vi "CorrectInvalidProfile.vi"(0 "v0x":dbl, 1 "s3x":dbl, 2 "s0x":dbl, 3 "a1":dbl, 4 "index":i32, 5 "v3x":dbl, 7 "Path  Smooth":dbl[][](array[numeric]), 9 "v3y":dbl, 11 "v0y":dbl, 12 "s3y":dbl, 13 "s0y":dbl, 14 "a3":dbl) -> (6 "New v3x":dbl, 10 "New v3y":dbl)   [LabVIEW 2018]
uses:
  <vilib>/Analysis/coordinate.llb/Wrap Angle (scalar).vi
  <vilib>/Analysis/_algsub.llb/Real Vector Norm.vi
  <vilib>/Analysis/NI_AAL_Angle.lvlib
  <vilib>/Analysis/NI_AALPro.lvlib
panel:
  out "v3x 2":dbl
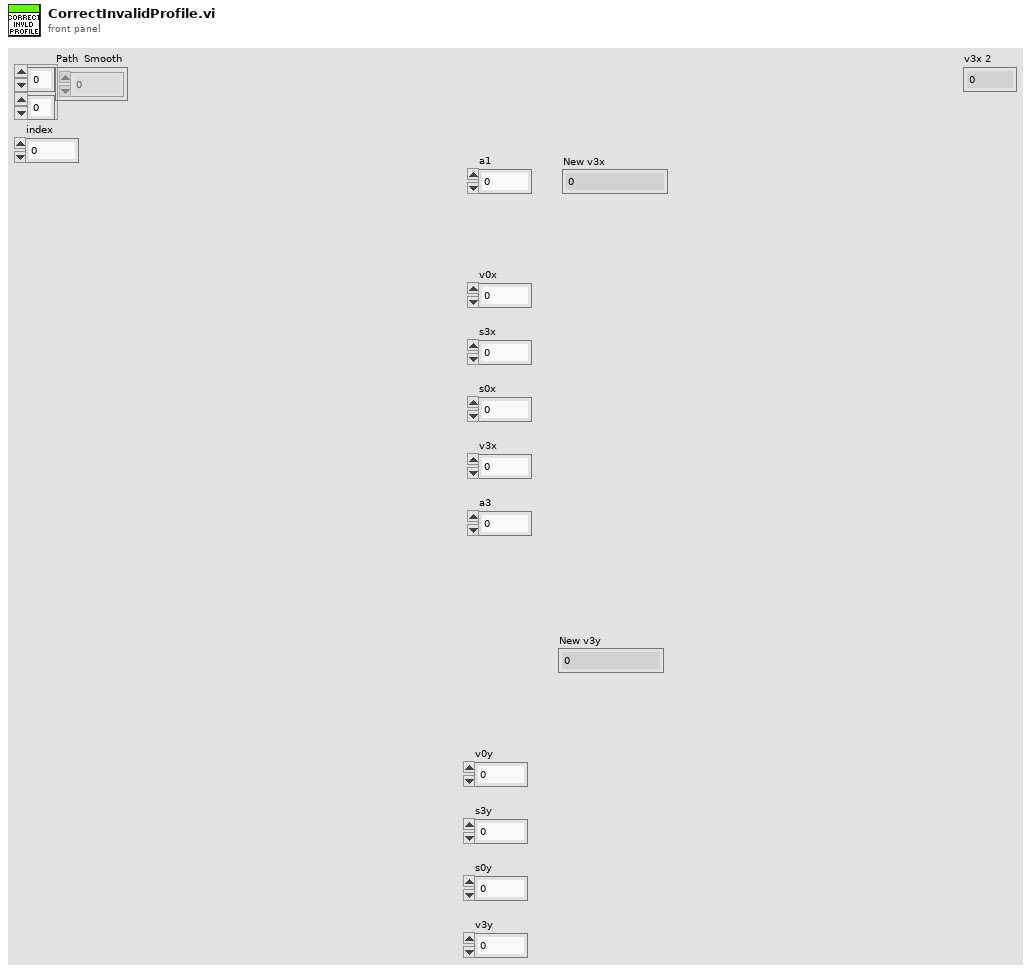
[diagram p1: front panel]
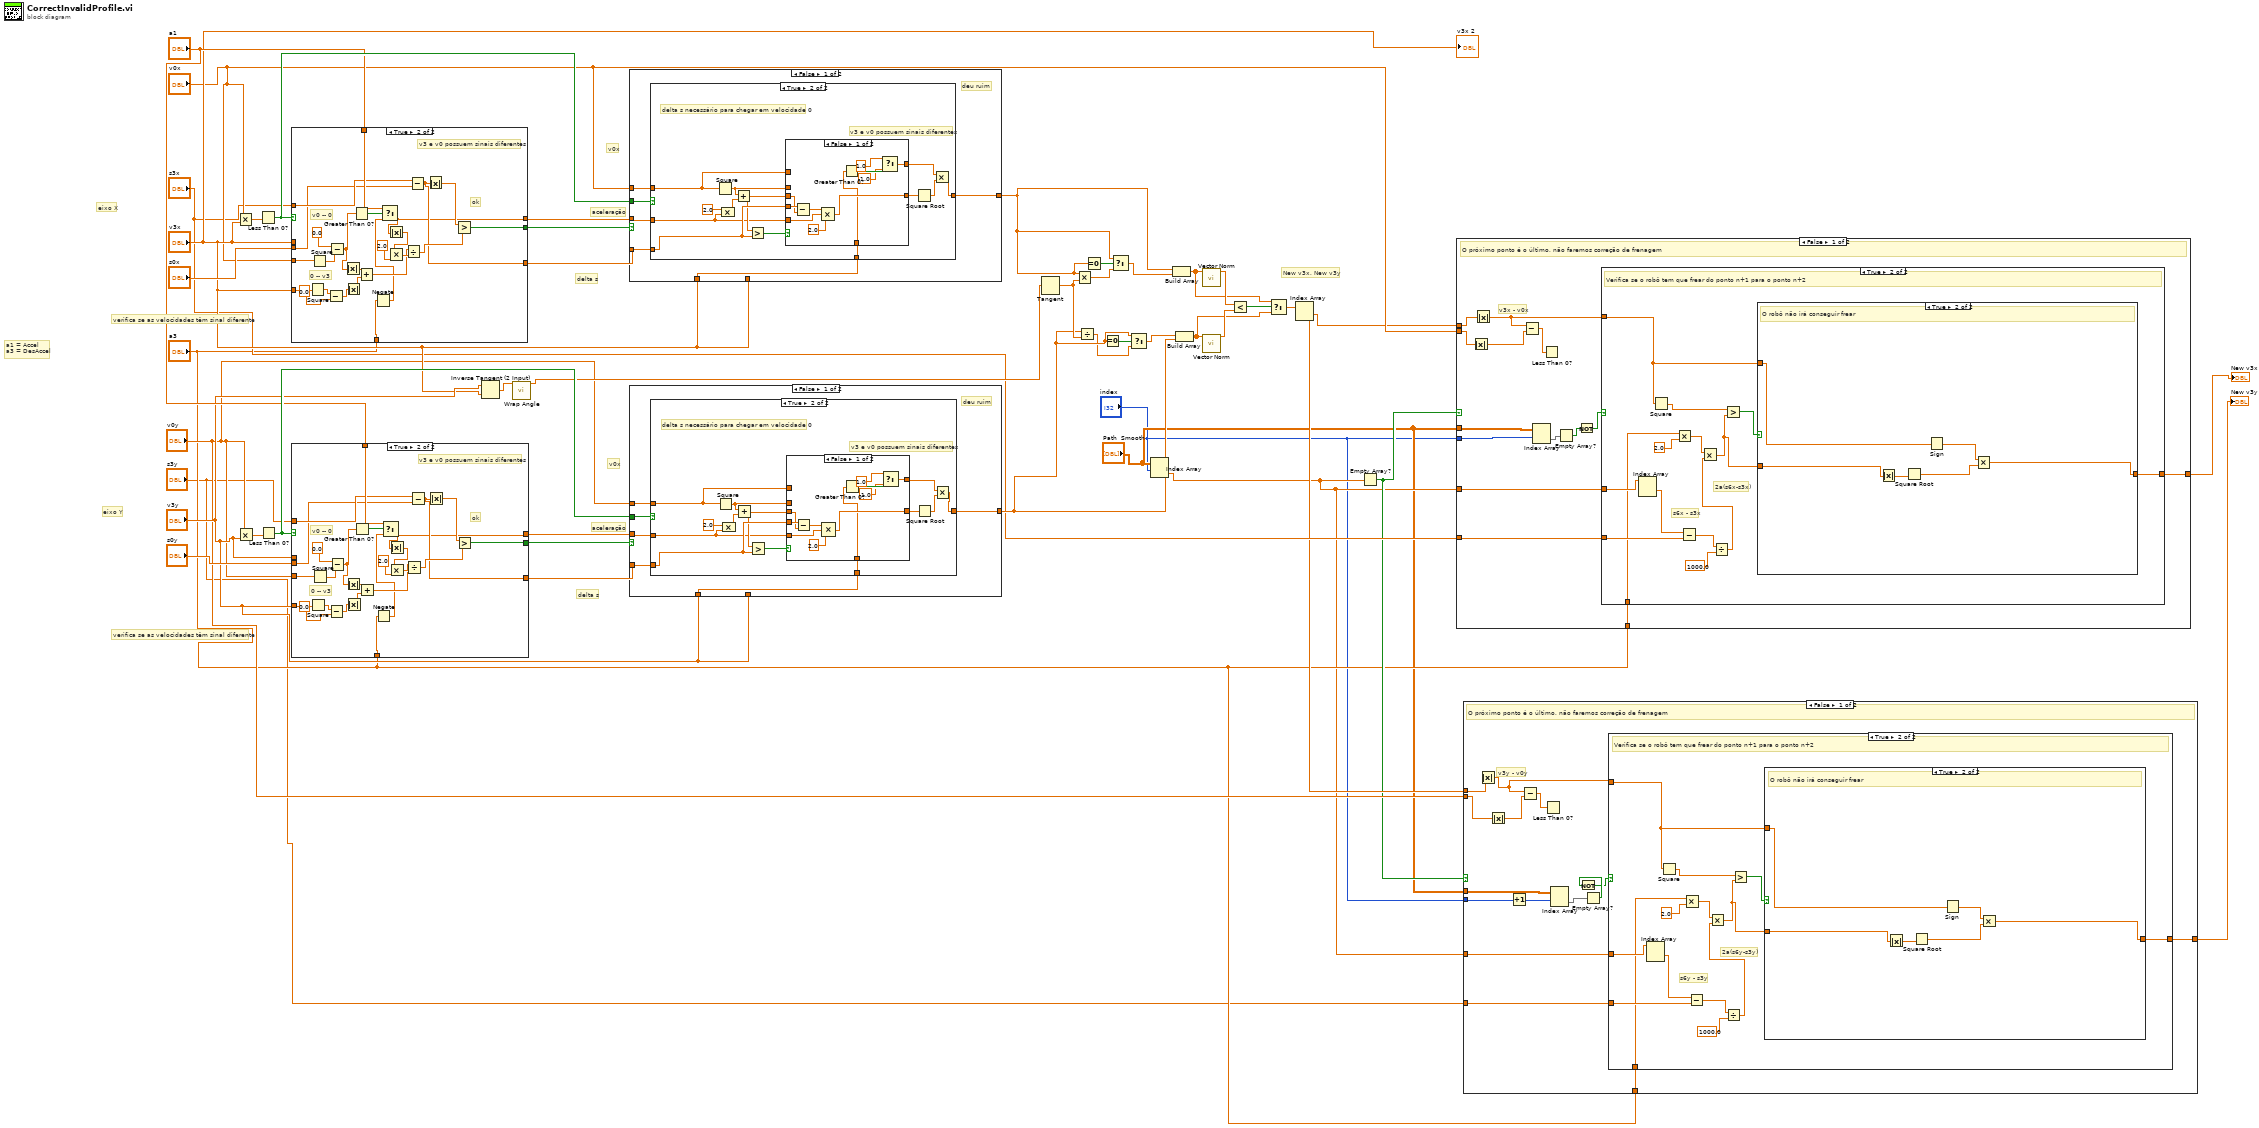
[diagram p0: block diagram]
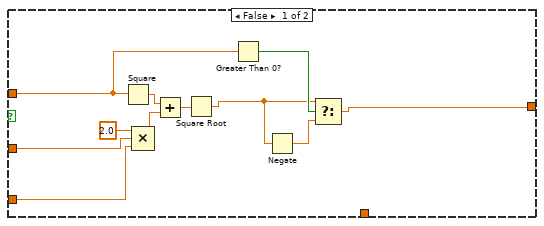
[diagram p8: hidden frame]
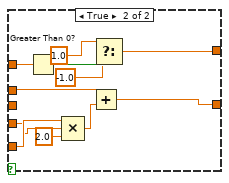
[diagram p9: hidden frame]
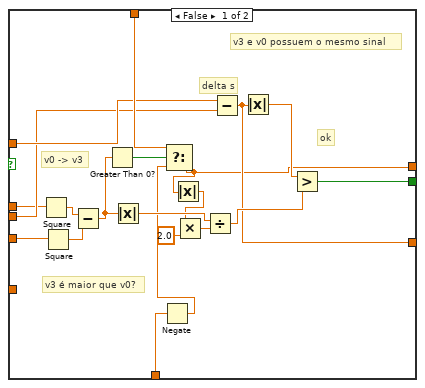
[diagram p11: hidden frame]
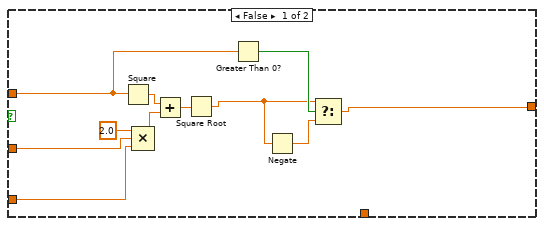
[diagram p12: hidden frame]
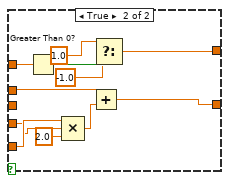
[diagram p13: hidden frame]
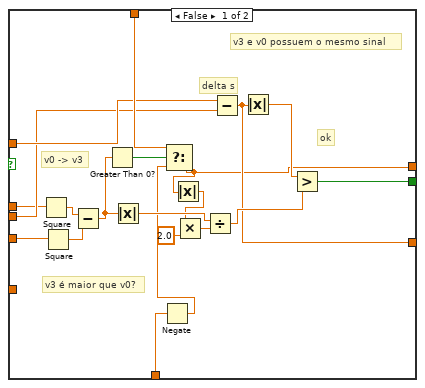
[diagram p15: hidden frame]
diagram:
  # "New v3x, New v3y"
  # "a1 = Accel\na3 = DesAccel"
  # "aceleração"
  # "v0x"
  # "verifica se as velocidades têm sinal diferente"
  # "delta s"
  # "aceleração"
  # "v0x"
  # "verifica se as velocidades têm sinal diferente"
  # "eixo Y"
  # "eixo X"
  # "delta s"
  n1 = Multiply(x="v0x", y="v3x") -> (x*y=w40:dbl)
  n2 = Multiply(x="v0y", y="v3y") -> (x*y=w35:dbl)
  n3 = Less Than 0?(x=w40) -> (x < 0?=w43:bool)
  n4 = Less Than 0?(x=w35) -> (x < 0?=w37:bool)
  n5 = case shown="True" w43 {
    tunnel: "v0x" -> [w63 w89]
    tunnel: "v3x" -> [_ w76]
    tunnel: "a3" -> [w49 w69]
    tunnel: "a1" -> [w59 w85]
    tunnel: "s3x" -> [w58 w84]
    tunnel: "s0x" -> [w57 w83]
    tunnel: [w54 w80] -> w42
    tunnel: "v3x" -> [w53 _]
    tunnel: [w47 w67] -> w44
    tunnel: [w50 w70] -> w45
    frame False {
      # "v3 é maior que v0?"
      # "v3 e v0 possuem o mesmo sinal"
      # "delta s"
      # "ok"
      # "v0 -> v3"
      n6 = Square(x=w53) -> (x^2=w65:dbl)
      n7 = Square(x=w63) -> (x^2=w64:dbl)
      n8 = Subtract(x=w65, y=w64) -> (x-y=w52:dbl)
      n9 = Greater Than 0?(x=w52) -> (x > 0?=w62:bool)
      n10 = Absolute Value(x=w52) -> (abs(x)=w51:dbl)
      n11 = Negate(x=w49) -> (-x=w48:dbl)
      n12 = Select(t=w59, s=w62, f=w48) -> (s? t:f=w47:dbl)
      n13 = Absolute Value(x=w47) -> (abs(x)=w46:dbl)
      n14 = Multiply(x=w46, y=2.0) -> (x*y=w61:dbl)
      n15 = Divide(x=w51, y=w61) -> (x/y=w55:dbl)
      n16 = Subtract(x=w58, y=w57) -> (x-y=w50:dbl)
      n17 = Absolute Value(x=w50) -> (abs(x)=w56:dbl)
      n18 = Greater?(x=w56, y=w55) -> (0:w54:bool)
    }
    frame True {
      # "v3 e v0 possuem sinais diferentes"
      # "0 -- v3"
      # "ok"
      # "v0 -- 0"
      n19 = Square(x=w76) -> (x^2=w79:dbl)
      n20 = Square(x=w89) -> (x^2=w90:dbl)
      n21 = Subtract(x=w79, y=0.0) -> (x-y=w72:dbl)
      n22 = Subtract(x=0.0, y=w90) -> (x-y=w74:dbl)
      n23 = Absolute Value(x=w74) -> (abs(x)=w73:dbl)
      n24 = Absolute Value(x=w72) -> (abs(x)=w71:dbl)
      n25 = Greater Than 0?(x=w74) -> (x > 0?=w88:bool)
      n26 = Add(x=w73, y=w71) -> (x+y=w75:dbl)
      n27 = Negate(x=w69) -> (-x=w68:dbl)
      n28 = Select(t=w85, s=w88, f=w68) -> (s? t:f=w67:dbl)
      n29 = Absolute Value(x=w67) -> (abs(x)=w66:dbl)
      n30 = Multiply(x=w66, y=2.0) -> (x*y=w87:dbl)
      n31 = Divide(x=w75, y=w87) -> (x/y=w81:dbl)
      n32 = Subtract(x=w84, y=w83) -> (x-y=w70:dbl)
      n33 = Absolute Value(x=w70) -> (abs(x)=w82:dbl)
      n34 = Greater?(x=w82, y=w81) -> (0:w80:bool)
    }
  }
  n35 = case shown="True" w37 {
    tunnel: "v0y" -> [w108 w134]
    tunnel: "v3y" -> [_ w121]
    tunnel: "a3" -> [w94 w114]
    tunnel: "a1" -> [w104 w130]
    tunnel: "s3y" -> [w103 w129]
    tunnel: "s0y" -> [w102 w128]
    tunnel: [w99 w125] -> w36
    tunnel: "v3y" -> [w98 _]
    tunnel: [w92 w112] -> w38
    tunnel: [w95 w115] -> w39
    frame False {
      # "v3 é maior que v0?"
      # "v3 e v0 possuem o mesmo sinal"
      # "delta s"
      # "ok"
      # "v0 -> v3"
      n36 = Square(x=w98) -> (x^2=w110:dbl)
      n37 = Square(x=w108) -> (x^2=w109:dbl)
      n38 = Subtract(x=w110, y=w109) -> (x-y=w97:dbl)
      n39 = Greater Than 0?(x=w97) -> (x > 0?=w107:bool)
      n40 = Absolute Value(x=w97) -> (abs(x)=w96:dbl)
      n41 = Negate(x=w94) -> (-x=w93:dbl)
      n42 = Select(t=w104, s=w107, f=w93) -> (s? t:f=w92:dbl)
      n43 = Absolute Value(x=w92) -> (abs(x)=w91:dbl)
      n44 = Multiply(x=w91, y=2.0) -> (x*y=w106:dbl)
      n45 = Divide(x=w96, y=w106) -> (x/y=w100:dbl)
      n46 = Subtract(x=w103, y=w102) -> (x-y=w95:dbl)
      n47 = Absolute Value(x=w95) -> (abs(x)=w101:dbl)
      n48 = Greater?(x=w101, y=w100) -> (0:w99:bool)
    }
    frame True {
      # "v3 e v0 possuem sinais diferentes"
      # "0 -- v3"
      # "ok"
      # "v0 -- 0"
      n49 = Square(x=w121) -> (x^2=w124:dbl)
      n50 = Square(x=w134) -> (x^2=w135:dbl)
      n51 = Subtract(x=w124, y=0.0) -> (x-y=w117:dbl)
      n52 = Subtract(x=0.0, y=w135) -> (x-y=w119:dbl)
      n53 = Absolute Value(x=w119) -> (abs(x)=w118:dbl)
      n54 = Absolute Value(x=w117) -> (abs(x)=w116:dbl)
      n55 = Greater Than 0?(x=w119) -> (x > 0?=w133:bool)
      n56 = Add(x=w118, y=w116) -> (x+y=w120:dbl)
      n57 = Negate(x=w114) -> (-x=w113:dbl)
      n58 = Select(t=w130, s=w133, f=w113) -> (s? t:f=w112:dbl)
      n59 = Absolute Value(x=w112) -> (abs(x)=w111:dbl)
      n60 = Multiply(x=w111, y=2.0) -> (x*y=w132:dbl)
      n61 = Divide(x=w120, y=w132) -> (x/y=w126:dbl)
      n62 = Subtract(x=w129, y=w128) -> (x-y=w115:dbl)
      n63 = Absolute Value(x=w115) -> (abs(x)=w127:dbl)
      n64 = Greater?(x=w127, y=w126) -> (0:w125:bool)
    }
  }
  n65 = Inverse Tangent (2 Input)(1:"v3x", 2:"v3y") -> (0:w31:dbl)
  n66 = call-poly <vilib>:"Wrap Angle.vi"("angle in"=w31) -> ("angle out"=w30:dbl)  [unwired: 9 in, 1 out]
  n67 = case shown="False" w42 {
    tunnel: w43 -> [w138 _]
    tunnel: "v0x" -> [w141 _]
    tunnel: w44 -> [w140 _]
    tunnel: w45 -> [w139 _]
    tunnel: [w137 w188] -> w21
    tunnel: "v3x" -> [_ w188]
    tunnel: "v3x" -> [w136 _]
    frame False {
      # "deu ruim"
      n68 = case shown="True" w138 {
        tunnel: w141 -> [w146 w157]
        tunnel: w140 -> [w149 w160]
        tunnel: w139 -> [w148 w162]
        tunnel: [w142 w154] -> w137
        tunnel: w136 -> [_ w153]
        frame False {
          n69 = Square(x=w146) -> (x^2=w152:dbl)
          n70 = Compound Arithmetic op=MULTIPLY(2.0 ("x"), w149, w148) -> (w151:dbl)
          n71 = Add(x=w152, y=w151) -> (x+y=w147:dbl)
          n72 = Square Root(x=w147) -> (sqrt(x)=w144:dbl)
          n73 = Greater Than 0?(x=w146) -> (x > 0?=w145:bool)
          n74 = Negate(x=w144) -> (-x=w143:dbl)
          n75 = Select(t=w144, s=w145, f=w143) -> (s? t:f=w142:dbl)
        }
        frame True {
          # "v3 e v0 possuem sinais diferentes"
          # "delta s necessário para chegar em velocidade 0"
          n76 = Square(x=w157) -> (x^2=w158:dbl)
          n77 = Compound Arithmetic op=MULTIPLY(2.0 ("x"), w160) -> (w165:dbl)
          n78 = Add(x=w158, y=w165) -> (x+y=w161:dbl)
          n79 = Greater?(x=w161, y=w162) -> (0:w163:bool)
          n80 = case shown="False" w163 {
            tunnel: w162 -> [w176 w184]
            tunnel: w161 -> [w175 _]
            tunnel: w160 -> [w173 w185]
            tunnel: [w171 w182] -> w159
            tunnel: w158 -> [_ w187]
            tunnel: w157 -> [_ w180]
            tunnel: [w167 w177] -> w156
            tunnel: w153 -> [w166 _]
            frame False {
              n81 = Subtract(x=w176, y=w175) -> (x-y=w174:dbl)
              n82 = Compound Arithmetic op=MULTIPLY(w174, w173, 2.0 ("value")) -> (w171:dbl)
              n83 = Greater Than 0?(x=w166) -> (x > 0?=w170:bool)
              n84 = Select(t=1.0, s=w170, f=-1.0) -> (s? t:f=w167:dbl)
            }
            frame True {
              n85 = Greater Than 0?(x=w180) -> (x > 0?=w181:bool)
              n86 = Compound Arithmetic op=MULTIPLY(w185, w184, 2.0 ("value")) -> (w186:dbl)
              n87 = Add(x=w187, y=w186) -> (x+y=w182:dbl)
              n88 = Select(t=1.0, s=w181, f=-1.0) -> (s? t:f=w177:dbl)
            }
          }
          n89 = Square Root(x=w159) -> (sqrt(x)=w155:dbl)
          n90 = Multiply(x=w156, y=w155) -> (x*y=w154:dbl)
        }
      }
    }
    frame True {
    }
  }
  n91 = case shown="False" w36 {
    tunnel: w37 -> [w191 _]
    tunnel: "v0y" -> [w194 _]
    tunnel: w38 -> [w193 _]
    tunnel: w39 -> [w192 _]
    tunnel: [w190 w241] -> w18
    tunnel: "v3y" -> [_ w241]
    tunnel: "v3y" -> [w189 _]
    frame False {
      # "deu ruim"
      n92 = case shown="True" w191 {
        tunnel: w194 -> [w199 w210]
        tunnel: w193 -> [w202 w213]
        tunnel: w192 -> [w201 w215]
        tunnel: [w195 w207] -> w190
        tunnel: w189 -> [_ w206]
        frame False {
          n93 = Square(x=w199) -> (x^2=w205:dbl)
          n94 = Compound Arithmetic op=MULTIPLY(2.0 ("x"), w202, w201) -> (w204:dbl)
          n95 = Add(x=w205, y=w204) -> (x+y=w200:dbl)
          n96 = Square Root(x=w200) -> (sqrt(x)=w197:dbl)
          n97 = Greater Than 0?(x=w199) -> (x > 0?=w198:bool)
          n98 = Negate(x=w197) -> (-x=w196:dbl)
          n99 = Select(t=w197, s=w198, f=w196) -> (s? t:f=w195:dbl)
        }
        frame True {
          # "v3 e v0 possuem sinais diferentes"
          # "delta s necessário para chegar em velocidade 0"
          n100 = Square(x=w210) -> (x^2=w211:dbl)
          n101 = Compound Arithmetic op=MULTIPLY(2.0 ("x"), w213) -> (w218:dbl)
          n102 = Add(x=w211, y=w218) -> (x+y=w214:dbl)
          n103 = Greater?(x=w214, y=w215) -> (0:w216:bool)
          n104 = case shown="False" w216 {
            tunnel: w215 -> [w229 w237]
            tunnel: w214 -> [w228 _]
            tunnel: w213 -> [w226 w238]
            tunnel: [w224 w235] -> w212
            tunnel: w211 -> [_ w240]
            tunnel: w210 -> [_ w233]
            tunnel: [w220 w230] -> w209
            tunnel: w206 -> [w219 _]
            frame False {
              n105 = Subtract(x=w229, y=w228) -> (x-y=w227:dbl)
              n106 = Compound Arithmetic op=MULTIPLY(w227, w226, 2.0 ("value")) -> (w224:dbl)
              n107 = Greater Than 0?(x=w219) -> (x > 0?=w223:bool)
              n108 = Select(t=1.0, s=w223, f=-1.0) -> (s? t:f=w220:dbl)
            }
            frame True {
              n109 = Greater Than 0?(x=w233) -> (x > 0?=w234:bool)
              n110 = Compound Arithmetic op=MULTIPLY(w238, w237, 2.0 ("value")) -> (w239:dbl)
              n111 = Add(x=w240, y=w239) -> (x+y=w235:dbl)
              n112 = Select(t=1.0, s=w234, f=-1.0) -> (s? t:f=w230:dbl)
            }
          }
          n113 = Square Root(x=w212) -> (sqrt(x)=w208:dbl)
          n114 = Multiply(x=w209, y=w208) -> (x*y=w207:dbl)
        }
      }
    }
    frame True {
    }
  }
  n115 = Tangent(1:w30) -> (0:w29:dbl)
  n116 = Multiply(x=w21, y=w29) -> (x*y=w20:dbl)
  n117 = Divide(x=w18, y=w29) -> (x/y=w17:dbl)
  n118 = Equal To 0?(x=w21) -> (x = 0?=w22:bool)
  n119 = Equal To 0?(x=w18) -> (x = 0?=w19:bool)
  n120 = Select(t=w21, s=w22, f=w20) -> (s? t:f=w15:dbl)
  n121 = Select(t=w18, s=w19, f=w17) -> (s? t:f=w16:dbl)
  n122 = Index Array(array="Path  Smooth", index (row)="index") -> (element=w3:dbl[])  [unwired: 1 in]
  n123 = Build Array(w21, w15) -> (w25:dbl[])
  n124 = Build Array(w16, w18) -> (w24:dbl[])
  n125 = call-poly <vilib>:"Vector Norm.vi"("Input Vector"=w24) -> ("norm"=w27:dbl)  [unwired: 9 in, 1 out]
  n126 = call-poly <vilib>:"Vector Norm.vi"("Input Vector"=w25) -> ("norm"=w28:dbl)  [unwired: 9 in, 1 out]
  n127 = Less?(x=w28, y=w27) -> (x < y?=w26:bool)
  n128 = Select(t=w25, s=w26, f=w24) -> (s? t:f=w23:dbl[])
  n129 = Index Array(array=w23) -> (element #1=w11:dbl, element #2=w9:dbl)  [unwired: 2 in]
  n130 = Empty Array?(array=w3) -> (empty?=w7:bool)
  n131 = case shown="False" w7 {
    tunnel: w11 -> [w249 w278]
    tunnel: "v0x" -> [w248 _]
    tunnel: w3 -> [w254 _]
    tunnel: "s3x" -> [w253 _]
    tunnel: "a3" -> [w252 _]
    tunnel: [w251 w278] -> w10
    tunnel: "index" -> [w242 _]
    tunnel: "Path  Smooth" -> [w246 _]
    frame False {
      # "v3x - v0x"
      # "O próximo ponto é o último, não faremos correção de frenagem"
      n132 = Absolute Value(x=w248) -> (abs(x)=w247:dbl)
      n133 = Absolute Value(x=w249) -> (abs(x)=w250:dbl)
      n134 = Subtract(x=w250, y=w247) -> (x-y=w255:dbl)
      n135 = Index Array(array=w246, index (row)=w242) -> (element=w245:dbl[])  [unwired: 1 in]
      n136 = Less Than 0?(x=w255) -> ()  [unwired: 1 out]
      n137 = Empty Array?(array=w245) -> (empty?=w244:bool)
      n138 = Not(x=w244) -> (.not. x?=w243:bool)
      n139 = case shown="True" w243 {
        tunnel: w254 -> [_ w269]
        tunnel: w253 -> [_ w268]
        tunnel: w252 -> [_ w266]
        tunnel: w250 -> [w256 w260]
        tunnel: [w256 w261] -> w251
        frame False {
          # "O robô não tem que frear, segue a vida normal"
        }
        frame True {
          # "2a(s6x-s3x)"
          # "s6x - s3x"
          # "Verifica se o robô tem que frear do ponto n+1 para o ponto n+2"
          n140 = Index Array(array=w269) -> (element #1=w270:dbl)  [unwired: 2 in, 1 out]
          n141 = Square(x=w260) -> (x^2=w264:dbl)
          n142 = Multiply(x=w266, y=2.0) -> (x*y=w267:dbl)
          n143 = Subtract(x=w270, y=w268) -> (x-y=w258:dbl)
          n144 = Divide(x=w258, y=1000.0) -> (x/y=w257:dbl)
          n145 = Multiply(x=w267, y=w257) -> (x*y=w262:dbl)
          n146 = Greater?(x=w264, y=w262) -> (0:w263:bool)
          n147 = case shown="True" w263 {
            tunnel: w262 -> [_ w277]
            tunnel: [w271 w272] -> w261
            tunnel: w260 -> [w271 w275]
            frame False {
              # "O robô irá conseguir frear"
            }
            frame True {
              # "O robô não irá conseguir frear"
              n148 = Absolute Value(x=w277) -> (abs(x)=w276:dbl)
              n149 = Square Root(x=w276) -> (sqrt(x)=w274:dbl)
              n150 = Sign(1:w275) -> (0:w273:dbl)
              n151 = Multiply(x=w273, y=w274) -> (x*y=w272:dbl)
            }
          }
        }
      }
    }
    frame True {
      # "Ativar correção de frenagem"
    }
  }
  "New v3x" <- w10
  n152 = case shown="False" w7 {
    tunnel: w9 -> [w288 w316]
    tunnel: "v0y" -> [w286 _]
    tunnel: w3 -> [w292 _]
    tunnel: "s3y" -> [w291 _]
    tunnel: "a3" -> [w290 _]
    tunnel: [w289 w316] -> w4
    tunnel: "Path  Smooth" -> [w282 _]
    tunnel: "index" -> [w281 _]
    frame False {
      # "v3y - v0y"
      # "O próximo ponto é o último, não faremos correção de frenagem"
      n153 = Absolute Value(x=w288) -> (abs(x)=w287:dbl)
      n154 = Absolute Value(x=w286) -> (abs(x)=w285:dbl)
      n155 = Increment(x=w281) -> (x+1=w284:i32)
      n156 = Subtract(x=w287, y=w285) -> (x-y=w293:dbl)
      n157 = Less Than 0?(x=w293) -> ()  [unwired: 1 out]
      n158 = Index Array(array=w282, index (row)=w284) -> (element=w283:dbl[])  [unwired: 1 in]
      n159 = Empty Array?(array=w283) -> (empty?=w280:bool)
      n160 = Not(x=w280) -> (.not. x?=w279:bool)
      n161 = case shown="True" w279 {
        tunnel: w292 -> [_ w307]
        tunnel: w291 -> [_ w306]
        tunnel: w290 -> [_ w304]
        tunnel: w287 -> [w294 w298]
        tunnel: [w294 w299] -> w289
        frame False {
          # "O robô não tem que frear, segue a vida normal"
        }
        frame True {
          # "2a(s6y-s3y)"
          # "s6y - s3y"
          # "Verifica se o robô tem que frear do ponto n+1 para o ponto n+2"
          n162 = Index Array(array=w307) -> (element #1=w308:dbl)  [unwired: 2 in, 1 out]
          n163 = Square(x=w298) -> (x^2=w302:dbl)
          n164 = Multiply(x=w304, y=2.0) -> (x*y=w305:dbl)
          n165 = Subtract(x=w308, y=w306) -> (x-y=w296:dbl)
          n166 = Divide(x=w296, y=1000.0) -> (x/y=w295:dbl)
          n167 = Multiply(x=w305, y=w295) -> (x*y=w300:dbl)
          n168 = Greater?(x=w302, y=w300) -> (0:w301:bool)
          n169 = case shown="True" w301 {
            tunnel: w300 -> [_ w315]
            tunnel: [w309 w310] -> w299
            tunnel: w298 -> [w309 w313]
            frame False {
              # "O robô irá conseguir frear"
            }
            frame True {
              # "O robô não irá conseguir frear"
              n170 = Absolute Value(x=w315) -> (abs(x)=w314:dbl)
              n171 = Square Root(x=w314) -> (sqrt(x)=w312:dbl)
              n172 = Sign(1:w313) -> (0:w311:dbl)
              n173 = Multiply(x=w311, y=w312) -> (x*y=w310:dbl)
            }
          }
        }
      }
    }
    frame True {
      # "Ativar correção de frenagem"
    }
  }
  "New v3y" <- w4
  "v3x 2" <- "v3x"
